vi "Write Tags.vi"(8 "error in (no error)":errorcluster, 11 "State in":T1={"State"=enum."Idle", "Start Time"=timestamp(0 s since 1904-01-01), "Configuration"={"Cycle Period"=0.0, "Setpoint Entry"=0.0, "Output Device"=enum."Huber Ministat 230", "Huber Ministat 230 Settings"={"VISA resource name"="", "Simulated?"=FALSE}, "Lauda Settings"={"VISA resource name"="", "Simulated?"=FALSE, "Pump Power"=2}, "Julabo FP-50 Settings"={"VISA resource name"="", "Simulated?"=FALSE, "Pump Power"=2}, "Internal Control?"=FALSE, "Huber Unistat 410 Settings"={"VISA resource name"="", "Simulated?"=FALSE}}, "Current Time"=timestamp(0 s since 1904-01-01), "First Iteration"=FALSE, "Data"={"TCU Speed"=0.0, "Temperature"=0.0}, "Process Name"="", "TCU On?"=FALSE, "Output Error"=FALSE, "Start Log"=FALSE, "Power Level Changed"=FALSE} {"Configuration"."Julabo FP-50 Settings"."Pump Power" min=0 max=8 step=1; "Configuration"."Lauda Settings"."Pump Power" min=0 max=8 step=1}) -> (0 "error out":errorcluster, 3 "State out":T1={"State"=enum."Idle", "Start Time"=timestamp(0 s since 1904-01-01), "Configuration"={"Cycle Period"=0.0, "Setpoint Entry"=0.0, "Output Device"=enum."Huber Ministat 230", "Huber Ministat 230 Settings"={"VISA resource name"="", "Simulated?"=FALSE}, "Lauda Settings"={"VISA resource name"="", "Simulated?"=FALSE, "Pump Power"=2}, "Julabo FP-50 Settings"={"VISA resource name"="", "Simulated?"=FALSE, "Pump Power"=2}, "Internal Control?"=FALSE, "Huber Unistat 410 Settings"={"VISA resource name"="", "Simulated?"=FALSE}}, "Current Time"=timestamp(0 s since 1904-01-01), "First Iteration"=FALSE, "Data"={"TCU Speed"=0.0, "Temperature"=0.0}, "Process Name"="", "TCU On?"=FALSE, "Output Error"=FALSE, "Start Log"=FALSE, "Power Level Changed"=FALSE} {"Configuration"."Julabo FP-50 Settings"."Pump Power" min=0 max=8 step=1; "Configuration"."Lauda Settings"."Pump Power" min=0 max=8 step=1})   [LabVIEW 2018, in "TCU Module.lvlib" / "TCU Module Engine.lvlib"]
uses:
  TCU Module Engine.lvlib
  TCU State Cluster.ctl
  State Enum.ctl
  TCU Module Settings Cluster.ctl
  Output Devices.ctl
  Huber TCU/Huber Settings.ctl
  Lauda Integral XT-150 TCU/Lauda Settings.ctl
  Julabo Type 1 TCU/Julabo Type 1 TCU Folder/Julabo FP-50 Settings.ctl
  Huber Unistat 410 TCU/Huber Unistat 410 Settings.ctl
  Tag VIs/Tag FGV Operation Enum.ctl
  Shared Variables/Dynamic Shared Variables.lvlib
  TCU Module.lvlib
  Huber TCU/Huber Ministat 230 TCU.lvlib
  Lauda Integral XT-150 TCU/Lauda TCU.lvlib
  Julabo Type 1 TCU/Julabo Type 1 TCU Folder/Julabo Type FP-50 TCU.lvlib
  Huber Unistat 410 TCU/Huber Unistat 410 TCU.lvlib
panel:
  # "Output Instruments"
  # "Output Instruments"
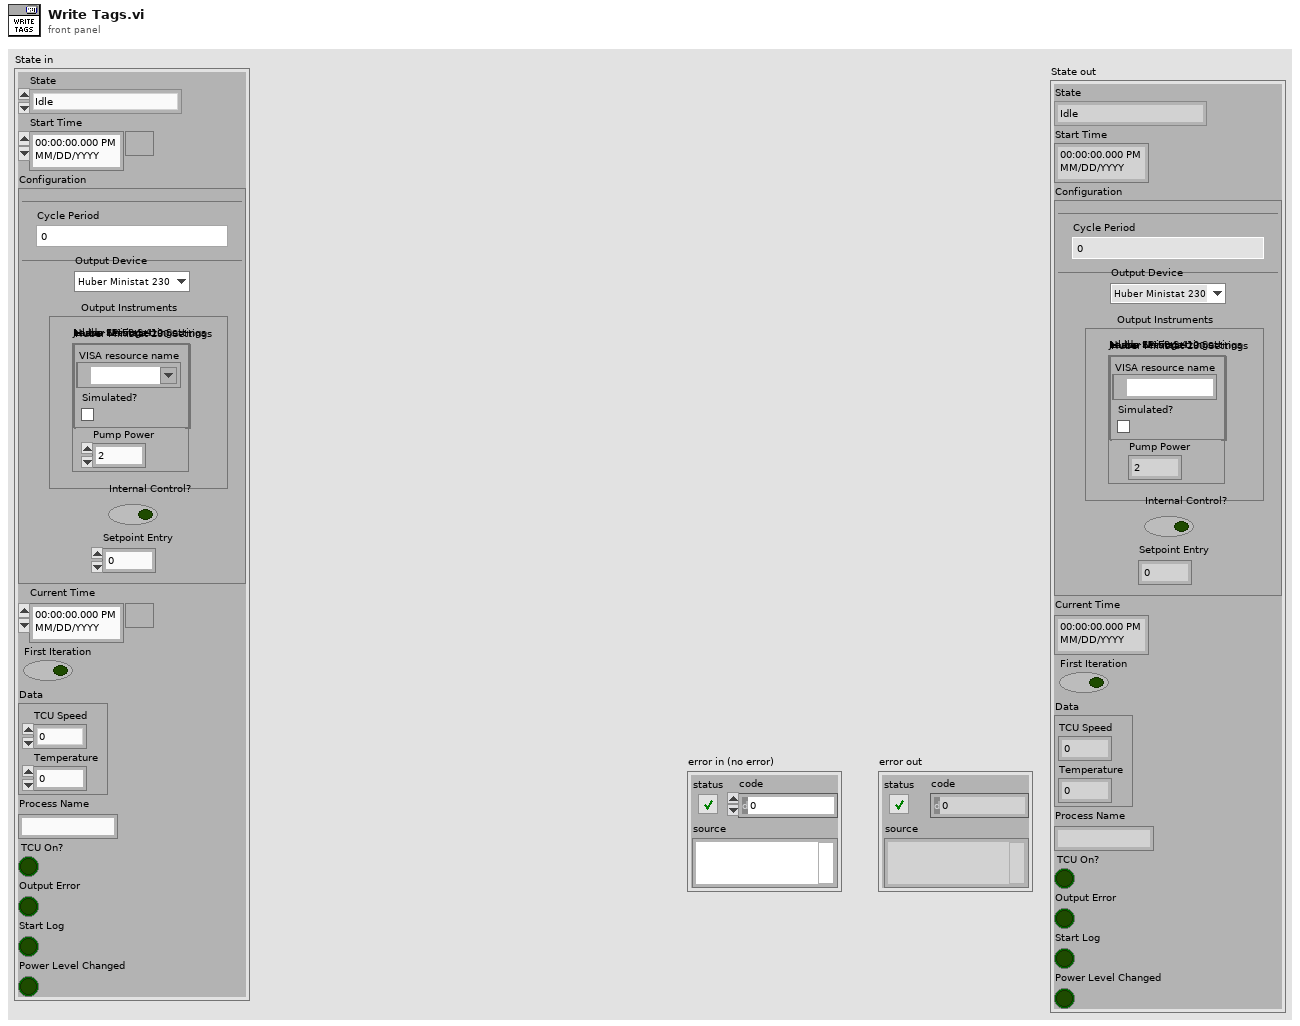
[diagram p1: front panel]
types:
  T1 = typedef "TCU Module.lvlib/TCU Module Engine.lvlib/TCU State Cluster.ctl" = cluster{"State":T2, "Start Time":timestamp, "Configuration":T3, "Current Time":timestamp, "First Iteration":bool, "Data":cluster{"TCU Speed":dbl, "Temperature":dbl}, "Process Name":string, "TCU On?":bool, "Output Error":bool, "Start Log":bool, "Power Level Changed":bool}
  T2 = typedef "TCU Module.lvlib/TCU Module Engine.lvlib/State Enum.ctl" = enum16{"Measuring", "Idle", "Paused"}
  T3 = typedef "TCU Module.lvlib/TCU Module Settings Cluster.ctl" = cluster{"Cycle Period":dbl, "Setpoint Entry":dbl, "Output Device":T4, "Huber Ministat 230 Settings":T5, "Lauda Settings":T6, "Julabo FP-50 Settings":T7, "Internal Control?":bool, "Huber Unistat 410 Settings":T8}
  T4 = typedef "Output Devices.ctl" = enum16{"Default", "Huber Ministat 230", "Huber Unistat 410", "Lauda XT-150", "Julabo FP-50"}
  T5 = typedef "Huber Ministat 230 TCU.lvlib/Huber Settings.ctl" = cluster{"VISA resource name":refnum<visa-resource-name>, "Simulated?":bool}
  T6 = typedef "Lauda TCU.lvlib/Lauda Settings.ctl" = cluster{"VISA resource name":refnum<visa-resource-name>, "Simulated?":bool, "Pump Power":i32}
  T7 = typedef "Julabo Type FP-50 TCU.lvlib/Julabo FP-50 Settings.ctl" = cluster{"VISA resource name":refnum<visa-resource-name>, "Simulated?":bool, "Pump Power":i32}
  T8 = typedef "Huber Unistat 410 TCU.lvlib/Huber Unistat 410 Settings.ctl" = cluster{"VISA resource name":refnum<visa-resource-name>, "Simulated?":bool}
  T9 = typedef "Tag FGV Operation Enum.ctl" = enum16{"Init", "Set Notification Queue", "Create Tag", "Commit", "Write Tag (Numeric)", "Write Tag (Boolean)", "Read All Tags", "Read One Tag", "Delete Tag Category", "Set Alarm Parameters (Numeric)", "Set Alarm Parameters (Boolean)", "Enable All Alarms", "Disable All Alarms", "Delete All Tags", "Read Alarms", "Ack Alarm", "Read Alarm Parameters (Numeric)", "Read Alarm Parameters (Boolean)"}
  T10 = typedef "TCU Module.lvlib/TCU Module Tag Names Cluster.ctl" = cluster{"TCU Temp":string, "Output Device Tag":string, "TCU Speed":string}
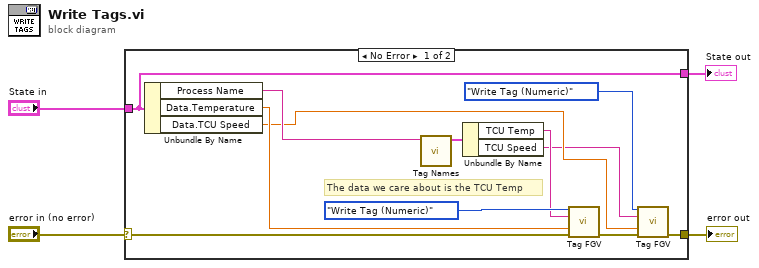
[diagram p0: block diagram]
diagram:
  n1 = case shown="No Error" "error in (no error)" {
    selector: "error in (no error)" -> [w11 w18]
    tunnel: [w5 w18] -> w3
    tunnel: "State in" -> [w14 w17]
    tunnel: [w14 w17] -> w1
    frame No Error {
      # "The data we care about is the TCU Temp"
      n2 = Unbundle By Name(w14) -> ("Process Name"=w16:string, "Data.Temperature"=w10:dbl, "Data.TCU Speed"=w7:dbl)
      n3 = call "Tag Names.vi"("Process Name"=w16) -> ("Pump Module Tag Names"=w13:T10)  [unwired: 8 in, 2 out]
      n4 = Unbundle By Name(w13) -> ("TCU Temp"=w12:string, "TCU Speed"=w6:string)
      n5 = call "Tag FGV.vi"("Operation"=Tag_FGV_Operation_Enum."Write Tag (Numeric)", "Tag Name"=w12, "Data"=w10, "error in (no error)"=w11) -> ("error out"=w8:errorcluster)  [unwired: 4 in, 7 out]
      n6 = call "Tag FGV.vi"("Operation"=Tag_FGV_Operation_Enum."Write Tag (Numeric)", "Tag Name"=w6, "Data"=w7, "error in (no error)"=w8) -> ("error out"=w5:errorcluster)  [unwired: 4 in, 7 out]
    }
    frame Error {
    }
  }
  "error out" <- w3
  "State out" <- w1
